vi "MaxFunktion.vi"(0 "VisaCluster":T2, 5 "Measurment":string, 7 "Max":T1, 11 "error in (no error)":errorcluster) -> (4 "VisaCluster 2":T2, 6 "Answer":string, 8 "Max 2":T1, 15 "error out":errorcluster)   [LabVIEW 2014, in "FH 55.lvlib"]
doc: "Dieses VI gibt die extremalen Messwerte aus dem Gerät zurück. Es kann zwischen keine Ausgabe, nur Max-Werte oder Max-Werte und Min-Werte gewählt werden.\n Durch die Taste Reset werden die extremalen Messwerte auf Null gesetzt. \n\n\nThis VI returns the extremal values from the instrument. You can choose between no output, only max values or max values and min values.\nWith the reset button, the extremal values are set to zero."
uses:
  FH 55.lvlib
  TypeDef/Max.ctl
  TypeDef/VisaCluster.ctl
  TypeDef/Value_String.ctl
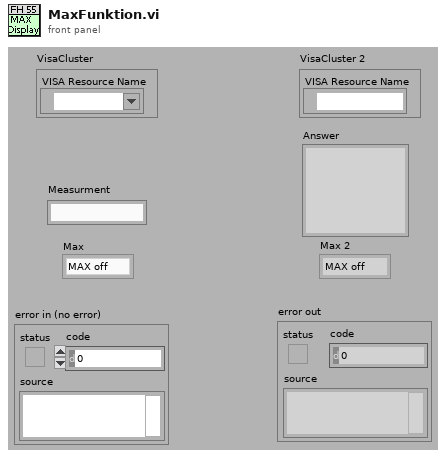
[diagram p1: front panel]
types:
  T1 = typedef "FH 55.lvlib/Max.ctl" = enum16{"MAX off", "Show MAX", "MAX/MIN"}
  T2 = typedef "FH 55.lvlib/VisaCluster.ctl" = cluster{"VISA Resource Name":refnum<visa-resource-name>}
  T3 = typedef "FH 55.lvlib/Value_String.ctl" = cluster{"Numeric":dbl, "String":string}
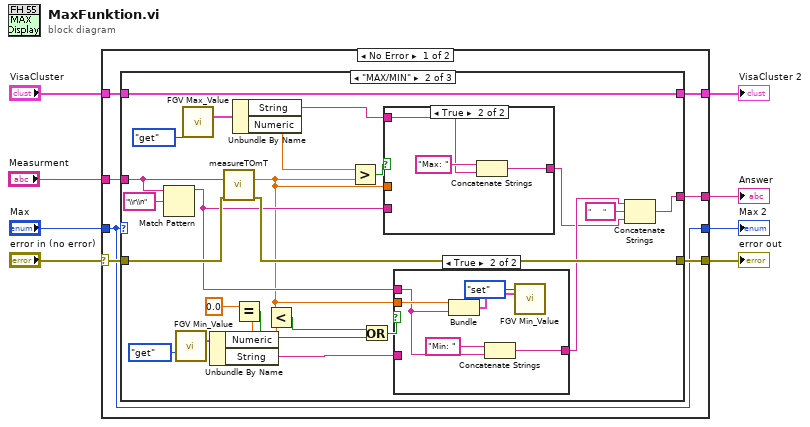
[diagram p0: block diagram]
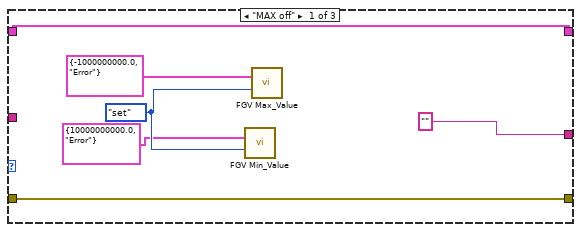
[diagram p2: hidden frame]
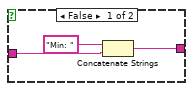
[diagram p3: hidden frame]
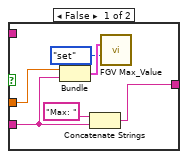
[diagram p4: hidden frame]
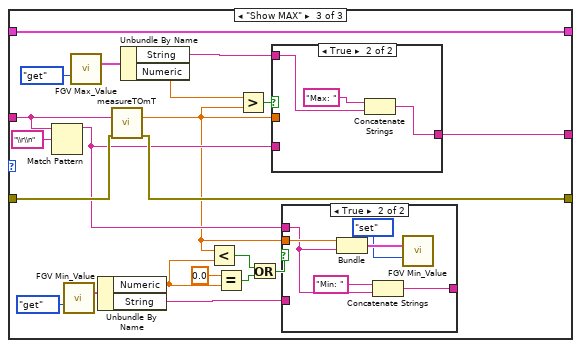
[diagram p5: hidden frame]
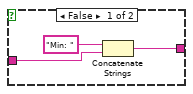
[diagram p6: hidden frame]
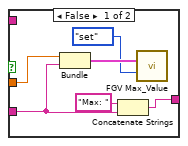
[diagram p7: hidden frame]
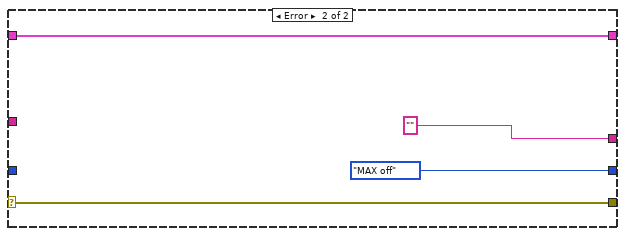
[diagram p8: hidden frame]
diagram:
  n1 = case shown="No Error" "error in (no error)" {
    selector: "error in (no error)" -> [w13 w105]
    tunnel: [w10 Max."MAX off" ("Max 2")] -> w8
    tunnel: [w15 "" ("Answer")] -> w7
    tunnel: "VisaCluster" -> [w14 w106]
    tunnel: "Max" -> [w10 _]
    tunnel: [w11 w106] -> w4
    tunnel: [w12 w105] -> w3
    tunnel: "Measurment" -> [w9 _]
    frame No Error {
      n2 = case shown="\"MAX/MIN\"" w10 {
        tunnel: w14 -> [w19 w40 w79]
        tunnel: ["" w33 w65] -> w15
        tunnel: w13 -> [w20 w39 w78]
        tunnel: [w20 w38 w77] -> w12
        tunnel: [w19 w40 w79] -> w11
        tunnel: w9 -> [_ w32 w73]
        frame "MAX off" {
          w17 = enum16{"set", "get"}."set" ("action")
          n3 = call "FGV Min_Value.vi"("Extrem_Value"=T3 {"Numeric"=10000000000.0, "String"="Error"}, "action"=w17) -> ()  [unwired: 13 in, 1 out]
          n4 = call "FGV Max_Value.vi"("Extrem_Value"=T3 {"Numeric"=-1000000000.0, "String"="Error"}, "action"=w17) -> ()  [unwired: 13 in, 1 out]
        }
        frame "MAX/MIN" {
          n5 = Match Pattern(string=w32, regular expression="\\r\\n") -> (before substring=w30:string)  [unwired: 1 in, 3 out]
          n6 = call "FGV Min_Value.vi"("action"=enum16{"set", "get"}."get") -> ("Extrem_Value 2"=w36:T3)  [unwired: 14 in]
          n7 = call "FGV Max_Value.vi"("action"=enum16{"set", "get"}."get") -> ("Extrem_Value 2"=w44:T3)  [unwired: 14 in]
          n8 = Unbundle By Name(w36) -> ("Numeric"=w28:dbl, "String"=w35:string)
          n9 = call "measureTOmT.vi"("string"=w32, "error in (no error)"=w39) -> ("Numeric"=w29:dbl, "error out"=w38:errorcluster)  [unwired: 11 in, 1 out]
          n10 = Unbundle By Name(w44) -> ("String"=w41:string, "Numeric"=w43:dbl)
          n11 = Equal?(x=0.0, y=w28) -> (x = y?=w26:bool)
          n12 = Less?(x=w29, y=w28) -> (x < y?=w25:bool)
          n13 = Greater?(x=w43, y=w29) -> (0:w42:bool)
          n14 = Or(x=w25, y=w26) -> (x .or. y?=w24:bool)
          n15 = case shown="True" w42 {
            tunnel: w30 -> [w57 _]
            tunnel: w41 -> [_ w61]
            tunnel: [w60 w62] -> w22
            tunnel: w29 -> [w58 _]
            frame False {
              n16 = Bundle("Numeric"=w58, "Measurment"=w57) -> (w56:cluster{"Numeric":dbl, "Measurment":string})  [unwired: 1 in]
              n17 = Concatenate Strings("Max: " ("string"), w57) -> (w60:string)
              n18 = call "FGV Max_Value.vi"("Extrem_Value"=w56, "action"=enum16{"set", "get"}."set") -> ()  [unwired: 13 in, 1 out]
            }
            frame True {
              n19 = Concatenate Strings("Max: " ("string"), w61) -> (w62:string)
            }
          }
          n20 = case shown="True" w24 {
            tunnel: w35 -> [w47 _]
            tunnel: [w46 w49] -> w23
            tunnel: w30 -> [_ w52]
            tunnel: w29 -> [_ w53]
            frame False {
              n21 = Concatenate Strings("Min: " ("string"), w47) -> (w46:string)
            }
            frame True {
              n22 = Bundle("Numeric"=w53, "Measurment"=w52) -> (w51:cluster{"Numeric":dbl, "Measurment":string})  [unwired: 1 in]
              n23 = Concatenate Strings("Min: " ("string"), w52) -> (w49:string)
              n24 = call "FGV Min_Value.vi"("Extrem_Value"=w51, "action"=enum16{"set", "get"}."set") -> ()  [unwired: 13 in, 1 out]
            }
          }
          n25 = Concatenate Strings(w23, "      " ("string"), w22) -> (w33:string)
        }
        frame "Show MAX" {
          n26 = Match Pattern(string=w73, regular expression="\\r\\n") -> (before substring=w71:string)  [unwired: 1 in, 3 out]
          n27 = call "FGV Min_Value.vi"("action"=enum16{"set", "get"}."get") -> ("Extrem_Value 2"=w75:T3)  [unwired: 14 in]
          n28 = call "FGV Max_Value.vi"("action"=enum16{"set", "get"}."get") -> ("Extrem_Value 2"=w83:T3)  [unwired: 14 in]
          n29 = Unbundle By Name(w75) -> ("Numeric"=w70:dbl, "String"=w74:string)
          n30 = call "measureTOmT.vi"("string"=w73, "error in (no error)"=w78) -> ("Numeric"=w64:dbl, "error out"=w77:errorcluster)  [unwired: 11 in, 1 out]
          n31 = Unbundle By Name(w83) -> ("String"=w80:string, "Numeric"=w82:dbl)
          n32 = Less?(x=w64, y=w70) -> (x < y?=w67:bool)
          n33 = Equal?(x=0.0, y=w70) -> (x = y?=w68:bool)
          n34 = Greater?(x=w82, y=w64) -> (0:w81:bool)
          n35 = Or(x=w67, y=w68) -> (x .or. y?=w66:bool)
          n36 = case shown="True" w81 {
            tunnel: w71 -> [w96 _]
            tunnel: w80 -> [_ w100]
            tunnel: [w99 w101] -> w65
            tunnel: w64 -> [w97 _]
            frame False {
              n37 = Bundle("Numeric"=w97, "Measurment"=w96) -> (w95:cluster{"Numeric":dbl, "Measurment":string})  [unwired: 1 in]
              n38 = Concatenate Strings("Max: " ("string"), w96) -> (w99:string)
              n39 = call "FGV Max_Value.vi"("Extrem_Value"=w95, "action"=enum16{"set", "get"}."set") -> ()  [unwired: 13 in, 1 out]
            }
            frame True {
              n40 = Concatenate Strings("Max: " ("string"), w100) -> (w101:string)
            }
          }
          n41 = case shown="True" w66 {
            tunnel: w74 -> [w86 _]
            tunnel: [w85 w88] -> _
            tunnel: w71 -> [_ w91]
            tunnel: w64 -> [_ w92]
            frame False {
              n42 = Concatenate Strings("Min: " ("string"), w86) -> (w85:string)
            }
            frame True {
              n43 = Bundle("Numeric"=w92, "Measurment"=w91) -> (w90:cluster{"Numeric":dbl, "Measurment":string})  [unwired: 1 in]
              n44 = Concatenate Strings("Min: " ("string"), w91) -> (w88:string)
              n45 = call "FGV Min_Value.vi"("Extrem_Value"=w90, "action"=enum16{"set", "get"}."set") -> ()  [unwired: 13 in, 1 out]
            }
          }
        }
      }
    }
    frame Error {
    }
  }
  "Max 2" <- w8
  "Answer" <- w7
  "error out" <- w3
  "VisaCluster 2" <- w4
